vi "writeToXML.vi"(8 "error in (no error)":errorcluster, 10 "ClassLabel":string, 11 "ProperMotion in":refnum<class "ProperMotion.lvclass">) -> (0 "error out":errorcluster, 2 "XMLout":string, 3 "ProperMotion out":refnum<class "ProperMotion.lvclass">)   [LabVIEW 2014, in "TCSDataDefinitions.lvlib" / "TCSCommand.lvlib" / "TargetConfiguration.lvlib" / "Target.lvlib" / "FixedTarget.lvlib" / "ProperMotion.lvclass"]
uses:
  ProperMotion.lvclass
  <userlib>/Common/UnitsAndXML/FlattenItemWithUnitToXML/FlattenAngularVelocityToXML/AngularVelocityUnit.ctl
  ProperMotion.lvclass/ProperMotion.ctl
  <userlib>/Common/UnitsAndXML/UnitsAndXML.lvlib
  <userlib>/Common/XML/XMLGenerator/XMLGenerator.lvclass
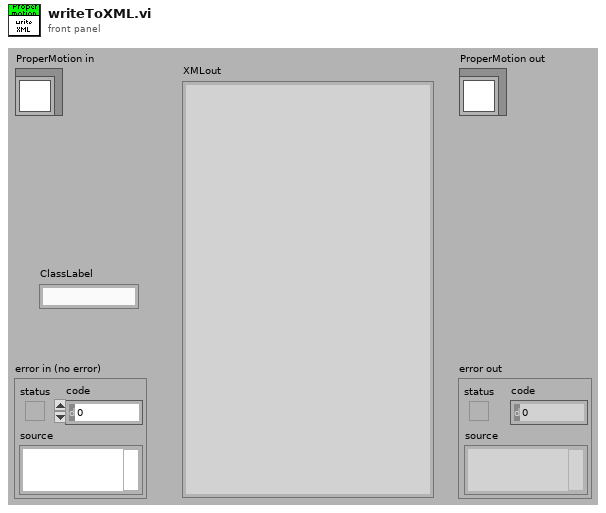
[diagram p1: front panel]
types:
  T1 = typedef "UnitsAndXML.lvlib/AngularVelocityUnit.ctl" = enum16{"\"/a", "deg/s", "\"/s"}
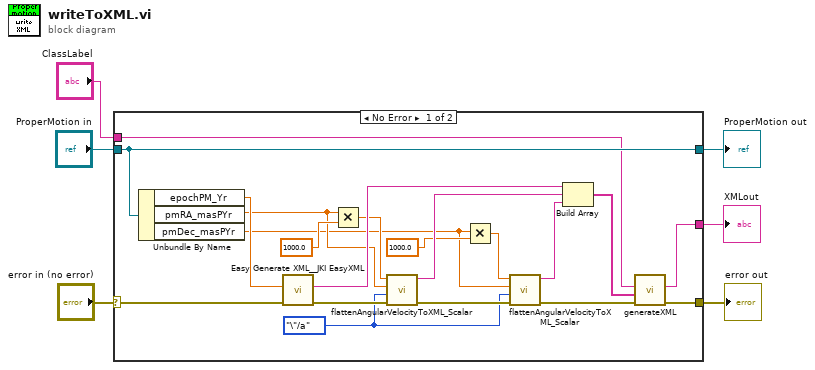
[diagram p0: block diagram]
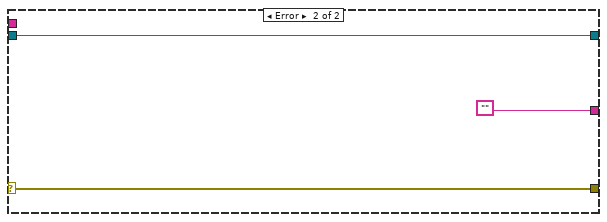
[diagram p2: hidden frame]
diagram:
  n1 = case shown="No Error" "error in (no error)" {
    selector: "error in (no error)" -> [w24 w29]
    tunnel: [w18 w29] -> w5
    tunnel: [w26 w28] -> w3
    tunnel: "ProperMotion in" -> [w26 w28]
    tunnel: "ClassLabel" -> [w19 _]
    tunnel: [w17 ""] -> w1
    frame No Error {
      w9 = AngularVelocityUnit."\"/a" ("angularVelocityUnitInXML")
      n2 = Unbundle By Name(w26) -> ("epochPM_Yr"=w25:dbl, "pmRA_masPYr"=w8:dbl[unit], "pmDec_masPYr"=w7:dbl[unit])
      n3 = call <vilib>:"Easy Generate XML__JKI EasyXML.vi"("error in (no error)"=w24, "LabVIEW Data"=w25) -> ("error out"=w23:errorcluster, "XML String"=w21:string)  [unwired: 8 in]
      n4 = Multiply(x=w8, y=1000.0) -> (x*y=w15:dbl[unit])
      n5 = call <userlib>:"flattenAngularVelocityToXML_Scalar.vi"("error in (no error)"=w23, "angularVelocityUnitInXML"=w9, "anuglarVelocityAgain"=w8, "angularVelocity"=w15) -> ("error out"=w14:errorcluster, "xmlString"=w22:string)  [unwired: 6 in]
      n6 = Multiply(x=w7, y=1000.0) -> (x*y=w11:dbl[unit])
      n7 = call <userlib>:"flattenAngularVelocityToXML_Scalar.vi"("error in (no error)"=w14, "angularVelocityUnitInXML"=w9, "anuglarVelocityAgain"=w7, "angularVelocity"=w11) -> ("error out"=w13:errorcluster, "xmlString"=w10:string)  [unwired: 6 in]
      n8 = Build Array(w21, w22, w10) -> (w20:string[])
      n9 = call <userlib>:"generateXML.vi"("error in"=w13, "childrenXML"=w20, "elementName"=w19) -> ("error out"=w18:errorcluster, "XML out"=w17:string)  [unwired: 6 in, 1 out]
    }
    frame Error {
    }
  }
  "error out" <- w5
  "ProperMotion out" <- w3
  "XMLout" <- w1
